vi "Data_Packets_To_Receiver_Table_Formatter.vi"(8 "error in (no error)":errorcluster, 11 "Data Packets In":T1[](array[typedef])) -> (0 "error out":errorcluster, 3 "Table contents":string[][](array[string]))   [LabVIEW 2017]
uses:
  Controls/Data Packets/Data_Packet.ctl
  Controls/Packet/Packet.ctl
  Controls/Packet/Packet_Direction.ctl
  Controls/Packet/Packet_Type.ctl
  Controls/Packet/Packet_Priority.ctl
  Controls/Data Packets/Parameter.ctl
  Controls/Data Packets/Parameter_Data_Type.ctl
  Controls/Data Packets/Data_Packet_Transmit_Mode.ctl
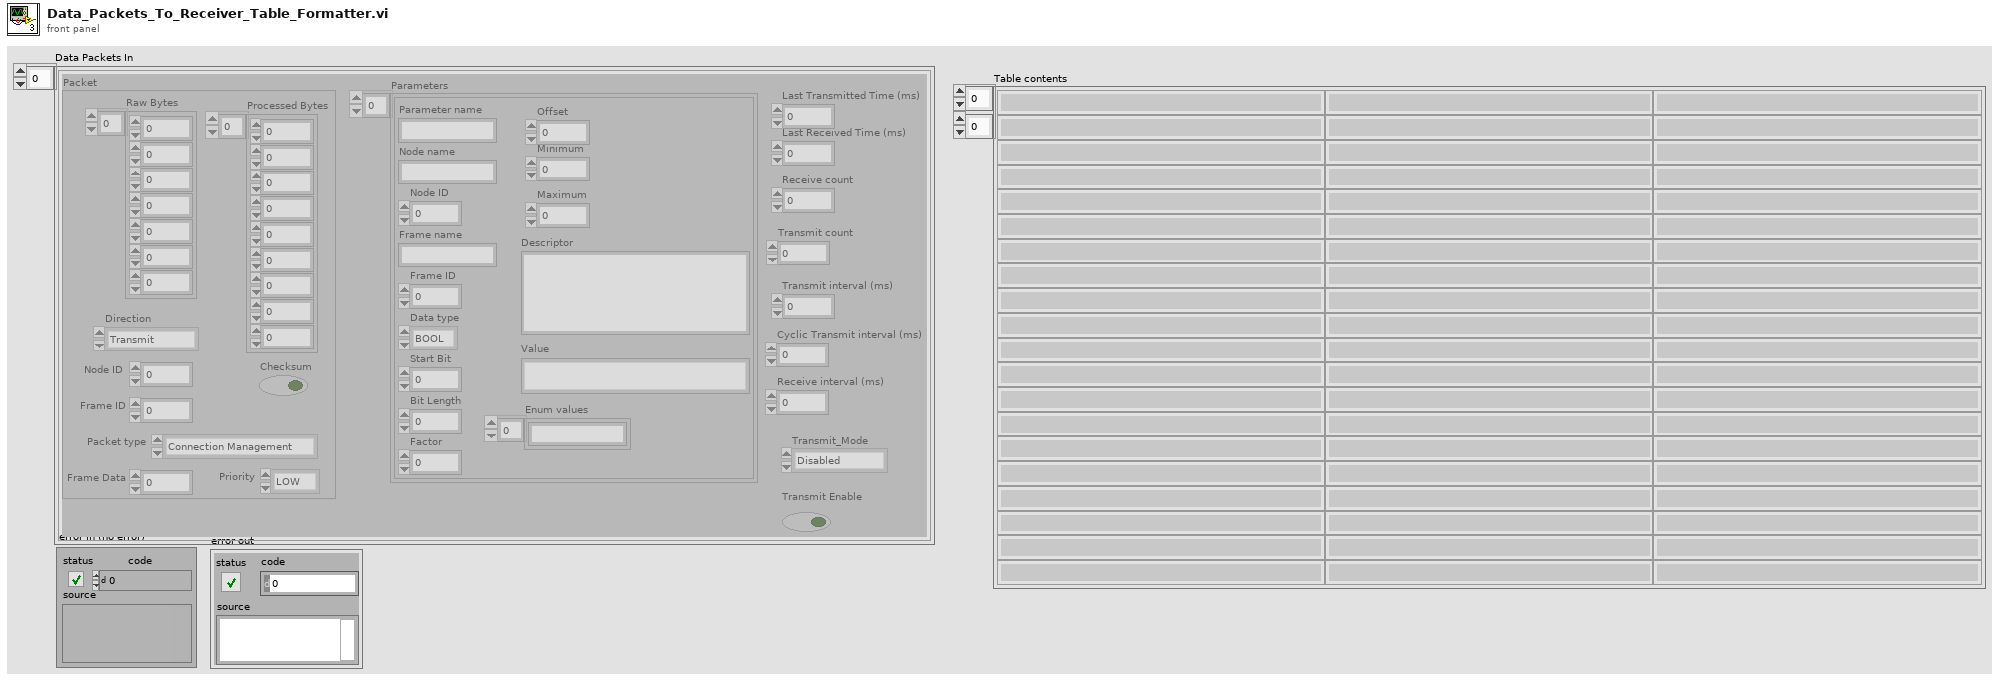
[diagram p1: front panel]
types:
  T1 = typedef "Data_Packet.ctl" = cluster{"Packet":T2, "Parameters":T6[], "Last Received Time (ms)":u64, "Receive count":i32, "Transmit count":i32, "Transmit interval (ms)":u32, "Last Transmitted Time (ms)":u64, "Receive interval (ms)":u32, "Transmit_Mode":T8, "Transmit Enable":bool, "Cyclic Transmit interval (ms)":u32}
  T2 = typedef "Packet.ctl" = cluster{"Raw Bytes":u8[], "Checksum":bool, "Direction":T3, "Processed Bytes":u8[], "Node ID":u8, "Packet type":T4, "Frame Data":u32, "Priority":T5, "Frame ID":u8}
  T3 = typedef "Packet_Direction.ctl" = enum16{"Transmit", "Receive", "Bidirectional"}
  T4 = typedef "Packet_Type.ctl" = enum16{"Data", "Connection Management", "Remote Request", "Error/Status"}
  T5 = typedef "Packet_Priority.ctl" = enum16{"LOW", "HIGH"}
  T6 = typedef "Parameter.ctl" = cluster{"Parameter name":string, "Node name":string, "Node ID":u8, "Frame name":string, "Frame ID":u8, "Data type":T7, "Start Bit":i32, "Bit Length":i32, "Factor":dbl, "Offset":dbl, "Minimum":dbl, "Maximum":dbl, "Descriptor":string, "Enum values":string[], "Value":string}
  T7 = typedef "Parameter_Data_Type.ctl" = enum16{"BOOL", "UNSIGNED", "SIGNED", "FLOAT32", "ENUM"}
  T8 = typedef "Data_Packet_Transmit_Mode.ctl" = enum16{"Disabled", "Single", "Cyclic"}
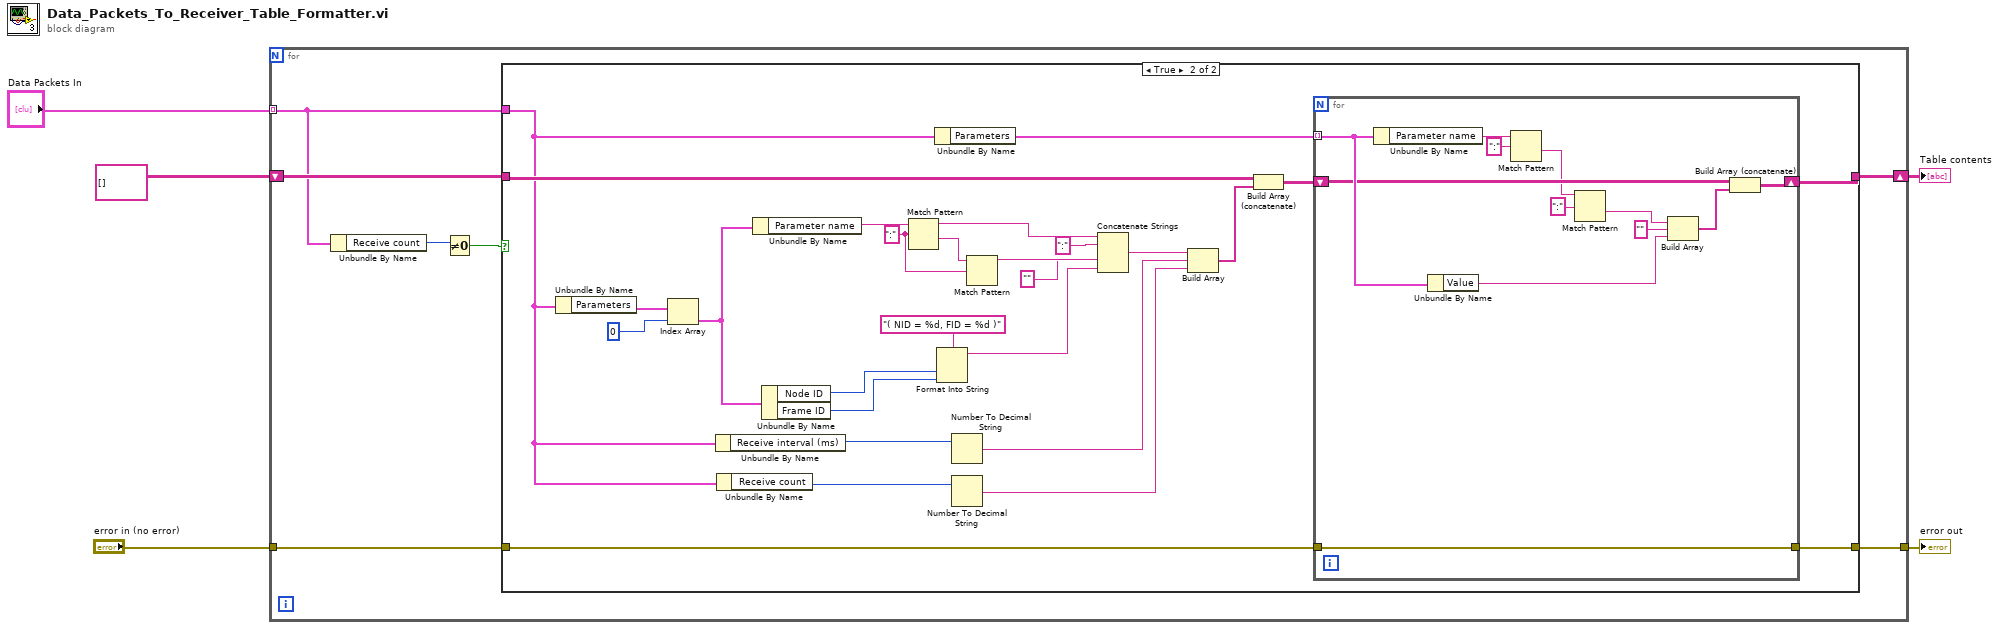
[diagram p0: block diagram]
diagram:
  n1 = for {
    tunnel: "Data Packets In" -> [w6] mode=indexing
    tunnel: "error in (no error)" -> [w11]
    tunnel: [w9] -> w2
    shift-right: [w7] -> w3
    shift-left: string[][] [] -> [w8]
    n2 = Unbundle By Name(w6) -> ("Receive count"=w12:i32)
    n3 = Not Equal To 0?(x=w12) -> (x != 0?=w10:bool)
    n4 = case shown="True" w10 {
      tunnel: w11 -> [w14 w16]
      tunnel: [w14 w15] -> w9
      tunnel: w8 -> [w13 w22]
      tunnel: [w13 w19] -> w7
      tunnel: w6 -> [_ w18]
      frame False {
      }
      frame True {
        w37 = ":" ("regular expression")
        n5 = Unbundle By Name(w18) -> ("Parameters"=w41:T6[])
        n6 = Index Array(array=w41, index=0) -> (element=w27:T6)
        n7 = Unbundle By Name(w18) -> ("Receive interval (ms)"=w26:u32)
        n8 = Unbundle By Name(w18) -> ("Receive count"=w24:i32)
        n9 = Unbundle By Name(w27) -> ("Parameter name"=w39:string)
        n10 = Unbundle By Name(w27) -> ("Node ID"=w30:u8, "Frame ID"=w29:u8)
        n11 = Match Pattern(string=w39, regular expression=w37) -> (before substring=w36:string, after substring=w38:string)  [unwired: 1 in, 2 out]
        n12 = Unbundle By Name(w18) -> ("Parameters"=w17:T6[])
        n13 = Format Into String(format string="( NID = %d, FID = %d )", w30, w29) -> (resulting string=w28:string)  [unwired: 2 in, 1 out]
        n14 = Number To Decimal String(number=w26) -> (decimal integer string=w25:string)  [unwired: 1 in]
        n15 = Number To Decimal String(number=w24) -> (decimal integer string=w23:string)  [unwired: 1 in]
        n16 = Match Pattern(string=w38, regular expression=w37) -> (before substring=w34:string)  [unwired: 1 in, 3 out]
        n17 = Concatenate Strings(w36, ":" ("string"), w34, "" ("string"), w28) -> (w33:string)
        n18 = Build Array(w33, w25, w23) -> (w21:string[])
        n19 = Build Array (concatenate)(w22, w21) -> (w20:string[][])
        n20 = for {
          shift-right: [w44] -> w19
          shift-left: w20 -> [w46]
          tunnel: w17 -> [w48] mode=indexing
          tunnel: w16 -> [w43]
          tunnel: [w43] -> w15
          n21 = Unbundle By Name(w48) -> ("Parameter name"=w53:string)
          n22 = Unbundle By Name(w48) -> ("Value"=w47:string)
          n23 = Match Pattern(string=w53, regular expression=":") -> (after substring=w42:string)  [unwired: 1 in, 3 out]
          n24 = Match Pattern(string=w42, regular expression=":") -> (after substring=w49:string)  [unwired: 1 in, 3 out]
          n25 = Build Array(w49, "", w47) -> (w45:string[])
          n26 = Build Array (concatenate)(w46, w45) -> (w44:string[][])
        }
      }
    }
  }
  "Table contents" <- w3
  "error out" <- w2
